vi "simple_scan_mathscript.vi"(0 "Piezo":dbl, 1 "Beam at max":dbl, 2 "Laser":i8, 3 "Sweep Interval":u32, 4 "Z mirror Gain":dbl, 5 "Sample Rate":i32, 6 "Z mirror offset":dbl, 7 "Sweep Time":u32, 8 "Z offset 2":dbl, 9 "Offset":dbl, 10 "Amplitude":dbl, 11 "Phase Shift":i32) -> ()   [LabVIEW 2013]
uses:
  <vilib>/DAQmx/create/channels.llb/DAQmx Create Channel (AO-Voltage-Basic).vi
  <vilib>/DAQmx/create/channels.llb/DAQmx Create Channel (DO-Digital Output).vi
  <vilib>/DAQmx/configure/timing.llb/DAQmx Timing (Sample Clock).vi
  <vilib>/DAQmx/write.llb/DAQmx Write (Analog 1D Wfm NChan NSamp).vi
  <vilib>/DAQmx/write.llb/DAQmx Write (Digital 1D Wfm NChan NSamp).vi
  <vilib>/Waveform/WDTOps.llb/WDT Number of Waveform Samples DBL.vi
  <vilib>/DAQmx/configure/trigger.llb/DAQmx Start Trigger (Digital Edge).vi
panel:
  out "output waveform":digitaldata
  out "Camera":digitalwaveform(graph)
  out "Z_mirror":waveform(dbl)(graph)
  out "Scan mirror":waveform(dbl)(graph)
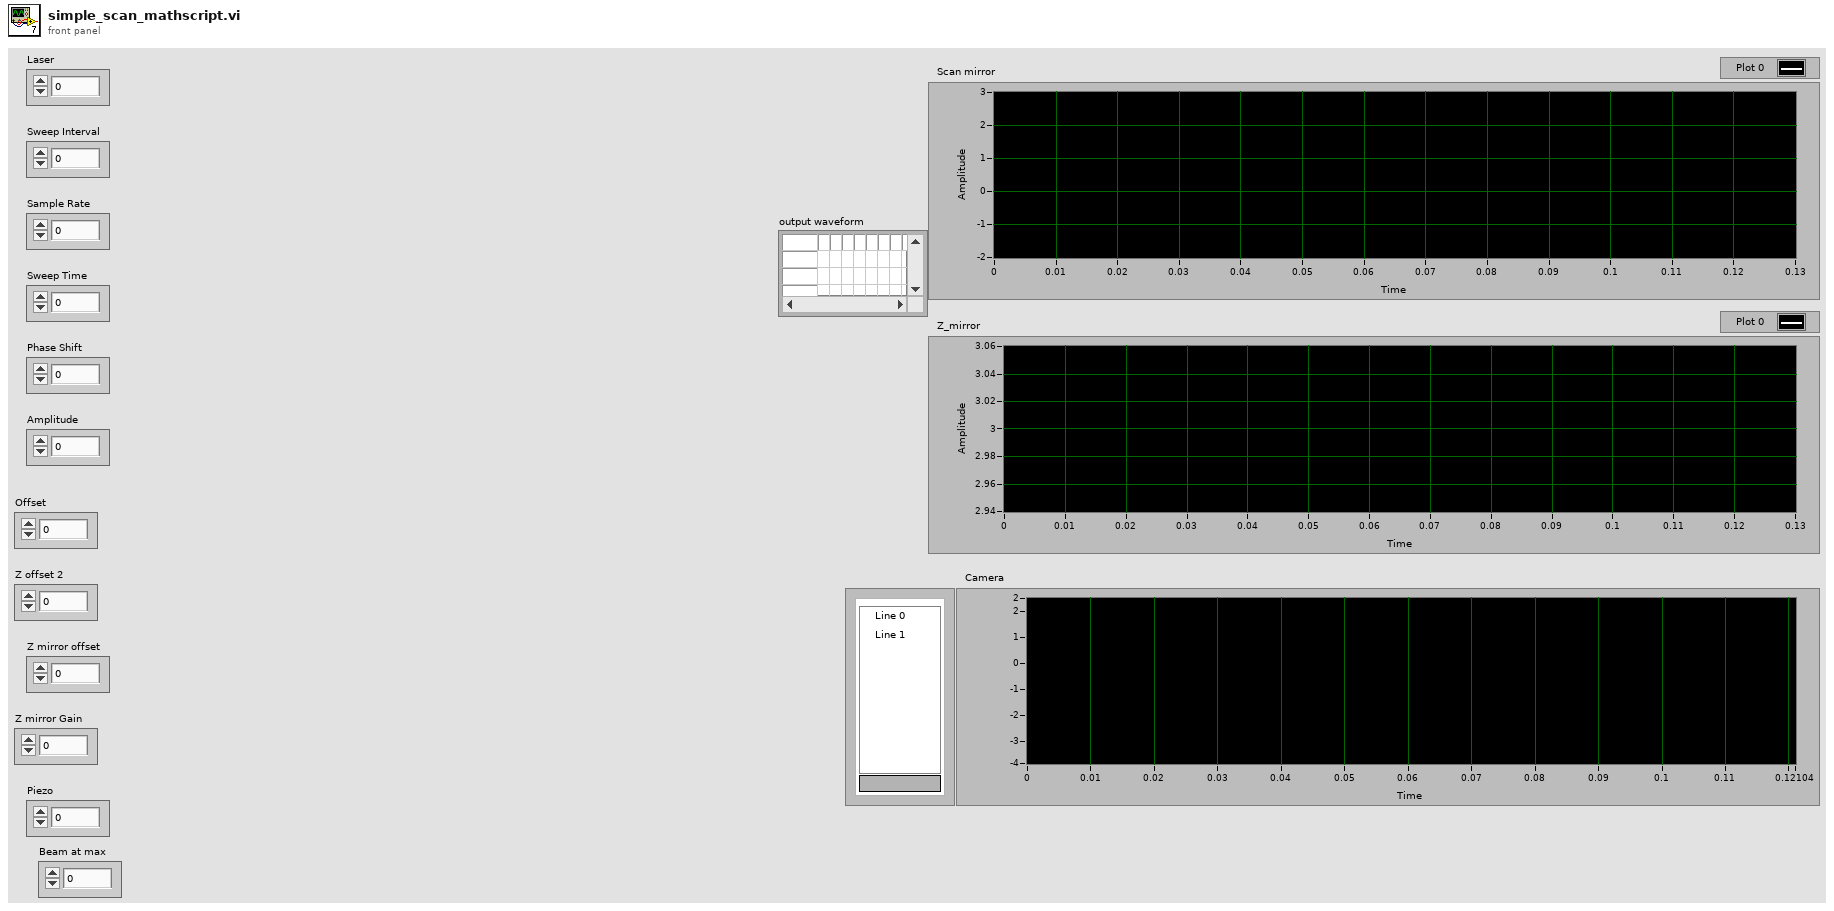
[diagram p1: front panel]
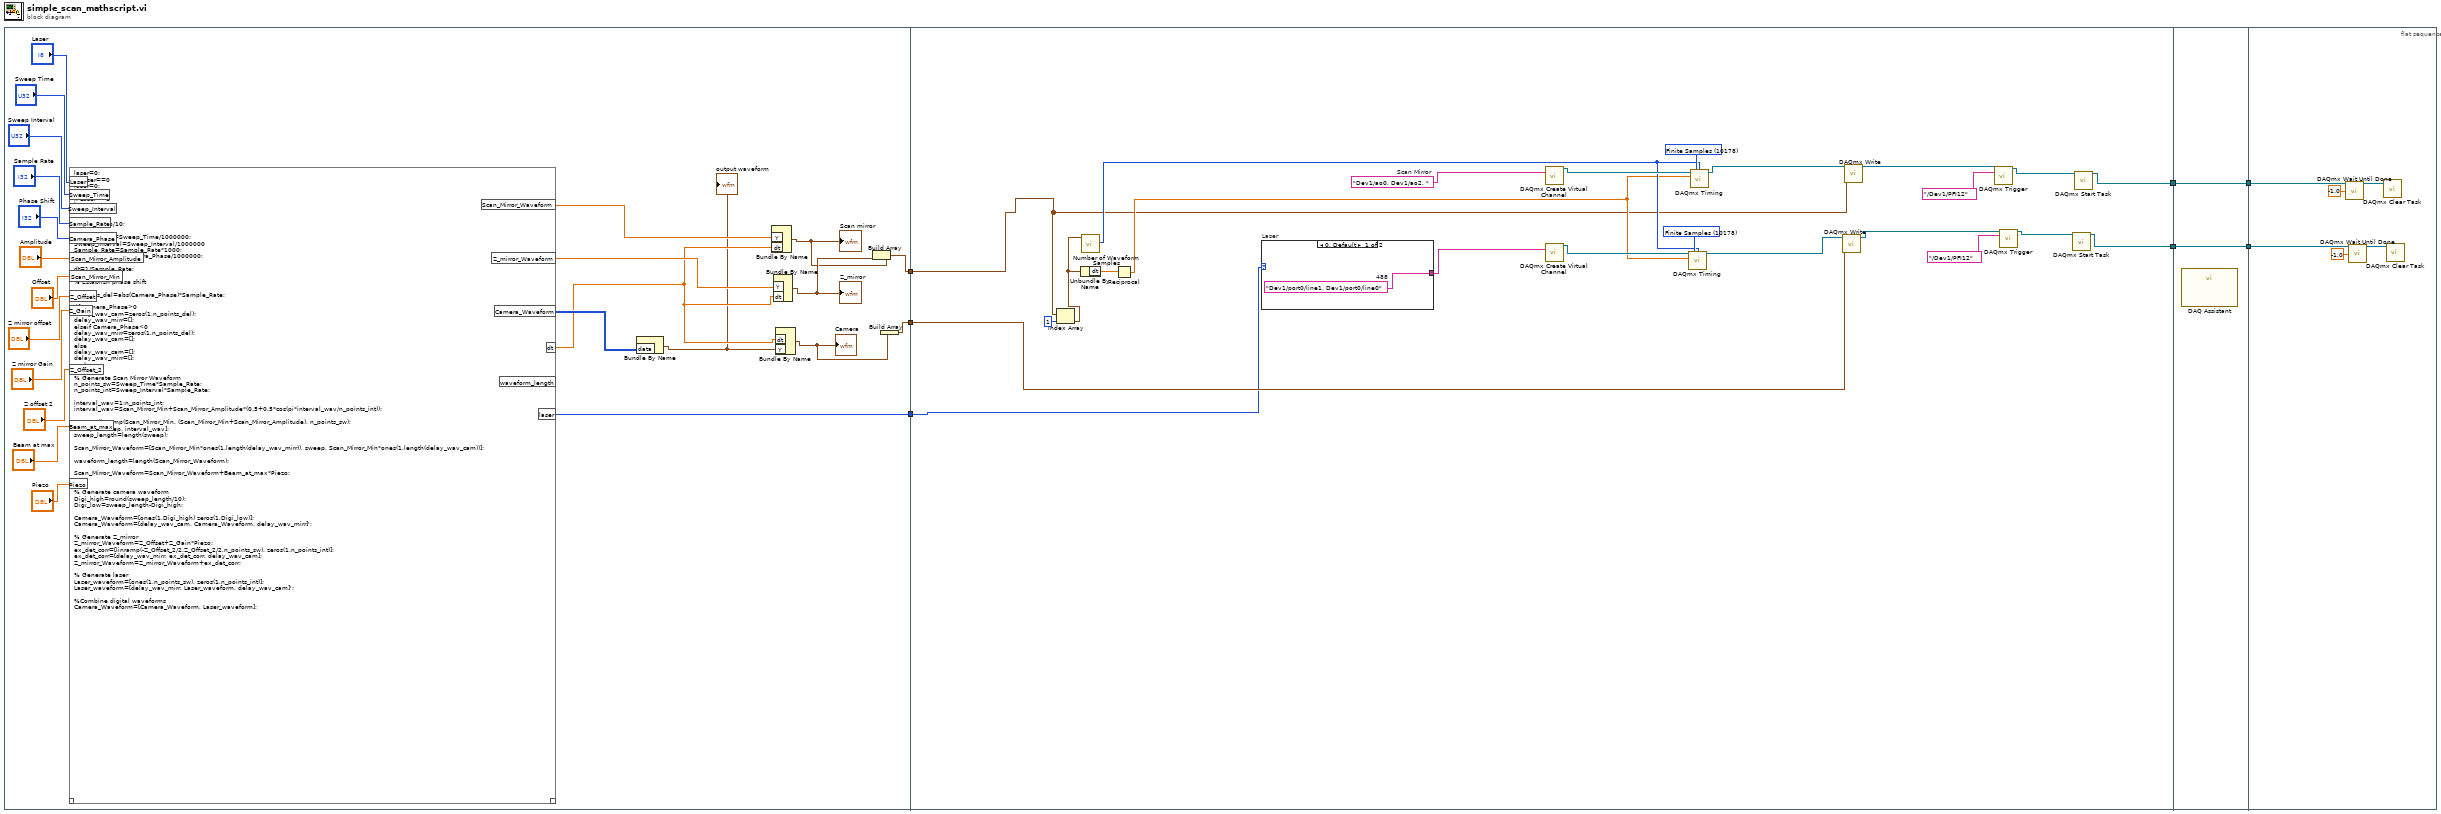
[diagram p0: block diagram]
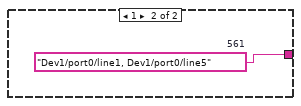
[diagram p2: hidden frame]
diagram:
  n1 = flat-sequence {
    tunnel: [w9] -> w3
    tunnel: [w10] -> w2
    tunnel: [w8] -> w1
    tunnel: [w40] -> w7
    tunnel: [w39] -> w6
    tunnel: w3 -> [w33]
    tunnel: w2 -> [w32]
    tunnel: w1 -> [w31]
    tunnel: [w58] -> w5
    tunnel: w7 -> [w58]
    tunnel: [w57] -> w4
    tunnel: w6 -> [w57]
    tunnel: w5 -> [w62]
    tunnel: w4 -> [w61]
    frame #0 {
      n2 = mathscript code="laser=0;\nif Laser==0\nlaser=0;\nend\nif Laser==1\nlaser=1;\nend\n\nPiezo=Piezo/10;\n\nSweep_Time=Sweep_Time/1000000;\nSweep_Interval=Sweep_Interval/1000000\nSample_Rate=Sample_Rate*1000;\nCamera_Phase=Camera_Phase/1000000;\n\ndt=1/Sample_Rate;\n\n% Establish phase shift\n\nn_points_del=abs(Camera_Phase)*Sample_Rate;\n\n if Camera_Phase>0\ndelay_wav_cam=zeros(1,n_points_del);\ndelay_wav_mirr=[];\nelseif Camera_Phase<0\ndelay_wav_mirr=zeros(1,n_points_del);\ndelay_wav_cam=[];\nelse\ndelay_wav_cam=[];\ndelay_wav_mirr=[];\nend\n\n% Generate Scan Mirror Waveform\nn_points_sw=Sweep_Time*Sample_Rate;\nn_points_int=Sweep_Interval*Sample_Rate;\n\ninterval_wav=1:n_points_int;\ninterval_wav=Scan_Mirror_Min+Scan_Mirror_Amplitude*(0.5+0.5*cos(pi*interval_wav/n_points_int));\n\nsweep=linramp(Scan_Mirror_Min, (Scan_Mirror_Min+Scan_Mirror_Amplitude), n_points_sw);\nsweep=[sweep, interval_wav];\nsweep_length=length(sweep);\n\nScan_Mirror_Waveform=[Scan_Mirror_Min*ones(1,length(delay_wav_mirr)), sweep, Scan_Mirror_Min*ones(1,length(delay_wav_cam))];\n\nwaveform_length=length(Scan_Mirror_Waveform);\n\nScan_Mirror_Waveform=Scan_Mirror_Waveform+Beam_at_max*Piezo;\n\n\n% Generate camera waveform\nDigi_high=round(sweep_length/10);\nDigi_low=sweep_length-Digi_high;\n\nCamera_Waveform=[ones(1,Digi_high) zeros(1,Digi_low)];\nCamera_Waveform=[delay_wav_cam, Camera_Waveform, delay_wav_mirr]';\n\n% Generate Z_mirror\nZ_mirror_Waveform=Z_Offset+Z_Gain*Piezo;\nex_det_corr=[linramp(-Z_Offset_2/2,Z_Offset_2/2,n_points_sw), zeros(1,n_points_int)];\nex_det_corr=[delay_wav_mirr, ex_det_corr, delay_wav_cam];\nZ_mirror_Waveform=Z_mirror_Waveform+ex_det_corr;\n\n% Generate laser\nLaser_waveform=[ones(1,n_points_sw), zeros(1,n_points_int)];\nLaser_waveform=[delay_wav_mirr, Laser_waveform, delay_wav_cam]';\n\n%Combine digital waveforms\nCamera_Waveform=[Camera_Waveform, Laser_waveform];"("Laser"="Laser", "Sweep_Time"="Sweep Time", "Sweep_Interval"="Sweep Interval", "Sample_Rate"="Sample Rate", "Camera_Phase"="Phase Shift", "Z_Offset"="Z mirror offset", "Scan_Mirror_Amplitude"="Amplitude", "Z_Gain"="Z mirror Gain", "Z_Offset_2"="Z offset 2", "Beam_at_max"="Beam at max", "Scan_Mirror_Min"="Offset", "Piezo"="Piezo") -> ("Scan_Mirror_Waveform"=w25:dbl[], "Z_mirror_Waveform"=w26:dbl[], "Camera_Waveform"=w27:i32[][], "dt"=w24:dbl, "laser"=w8:i32)  [unwired: 1 in, 2 out]
      n3 = Bundle By Name("data"=w27) -> (w23:digitaldata)  [unwired: 1 in]
      "output waveform" <- w23
      n4 = Bundle By Name ("Build Waveform")("Y"=w25, "dt"=w24) -> (w29:waveform(dbl))  [unwired: 1 in]
      "Scan mirror" <- w29
      n5 = Bundle By Name("Y"=w26, "dt"=w24) -> (w30:waveform(dbl))  [unwired: 1 in]
      "Z_mirror" <- w30
      n6 = Bundle By Name("dt"=w24, "Y"=w23) -> (w28:digitalwaveform)  [unwired: 1 in]
      "Camera" <- w28
      n7 = Build Array(w29, w30) -> (w10:waveform(dbl)[])
      n8 = Build Array(w28) -> (w9:digitalwaveform[])
    }
    frame #1 {
      w52 = 10178 items=["Finite Samples"=10178, "Continuous Samples"=10123, "Hardware Timed Single Point"=12522] ("sample mode")
      w53 = 10178 items=["Finite Samples"=10178, "Continuous Samples"=10123, "Hardware Timed Single Point"=12522] ("sample mode")
      w54 = tag "Dev1/ao0, Dev1/ao2, "  # Scan Mirror
      n9 = Index Array(array=w32, index=1) -> (element=w37:waveform(dbl))
      n10 = Unbundle By Name(w37) -> ("dt"=w47:dbl)
      n11 = call-poly <vilib>:"Number of Waveform Samples.vi"("waveform in"=w37) -> ("number of samples"=w36:i32)  [unwired: 8 in, 2 out]
      n12 = Reciprocal(x=w47) -> (1/x=w35:dbl)
      n13 = case "Laser" shown="0, Default" w31 {
        tunnel: [w55 w56] -> w34
        frame 0, Default {
          w55 = tag "Dev1/port0/line1, Dev1/port0/line0"  # 488
        }
        frame 1 {
          w56 = tag "Dev1/port0/line1, Dev1/port0/line5"  # 561
        }
      }
      n14 = call-poly <vilib>:"DAQmx Create Virtual Channel.vi"("physical channels"=w54) -> ("task out"=w51:refnum<k21>)  [unwired: 13 in, 1 out]
      n15 = call-poly <vilib>:"DAQmx Create Virtual Channel.vi"("lines"=w34) -> ("task out"=w50:refnum<k21>)  [unwired: 13 in, 1 out]
      n16 = call-poly <vilib>:"DAQmx Timing.vi"("task/channels in"=w50, "sample mode"=w52, "samples per channel"=w36, "rate"=w35) -> ("task out"=w48:refnum<k21>)  [unwired: 10 in, 1 out]
      n17 = call-poly <vilib>:"DAQmx Timing.vi"("task/channels in"=w51, "sample mode"=w53, "samples per channel"=w36, "rate"=w35) -> ("task out"=w49:refnum<k21>)  [unwired: 10 in, 1 out]
      n18 = call-poly <vilib>:"DAQmx Write.vi"("task/channels in"=w48, "data"=w33) -> ("task out"=w43:refnum<k21>)  [unwired: 3 in, 10 out]
      n19 = call-poly <vilib>:"DAQmx Write.vi"("task/channels in"=w49, "data"=w32) -> ("task out"=w44:refnum<k21>)  [unwired: 3 in, 10 out]
      n20 = call-poly <vilib>:"DAQmx Trigger.vi"("task/channels in"=w44, "source"=tag "/Dev1/PFI12") -> ("task out"=w42:refnum<k21>)  [unwired: 12 in, 1 out]
      n21 = call-poly <vilib>:"DAQmx Trigger.vi"("task/channels in"=w43, "source"=tag "/Dev1/PFI12") -> ("task out"=w41:refnum<k21>)  [unwired: 12 in, 1 out]
      n22 = call <vilib>:"DAQmx Start Task.vi"("task/channels in"=w41) -> ("task out"=w39:refnum<k21>)  [unwired: 1 in, 13 out]
      n23 = call <vilib>:"DAQmx Start Task.vi"("task/channels in"=w42) -> ("task out"=w40:refnum<k21>)  [unwired: 1 in, 13 out]
    }
    frame #2 {
      n24 = call "DAQ Assistant"() -> ()  [unwired: 18 in, 2 out]
    }
    frame #3 {
      n25 = call <vilib>:"DAQmx Wait Until Done.vi"("task/channels in"=w62, "timeout (sec)"=-1.0) -> ("task out"=w64:refnum<k21>)  [unwired: 12 in, 1 out]
      n26 = call <vilib>:"DAQmx Wait Until Done.vi"("task/channels in"=w61, "timeout (sec)"=-1.0) -> ("task out"=w63:refnum<k21>)  [unwired: 12 in, 1 out]
      n27 = call <vilib>:"DAQmx Clear Task.vi"("task in"=w64) -> ()  [unwired: 1 in, 14 out]
      n28 = call <vilib>:"DAQmx Clear Task.vi"("task in"=w63) -> ()  [unwired: 1 in, 14 out]
    }
  }
